vi "Bumper Start BAP7.vi"(11 "Port (Port 1)":T2=1 items=["Port 1", "Port 2", "Port 3", "Port 4"]) -> (3 "BrickReference out":T1)   [LabVIEW 2014]
doc: "Bumper Start BAP7\n\nPlays a note when front sensor is pressed. (Idle State)\n\nBeverly Abadines\nPHY 350\nBAP7"
uses:
  <vilib>/NXT/Block Support/NXT_InputPort.ctl
  <vilib>/NXT/Subs/LVHSConnector.ctl
  <vilib>/NXT/LegoClasses/BrickReference/BrickReference.lvclass
  <vilib>/NXT/Dual Mode Library/Sound/PlayC.vi
panel:
  # "Bumper Start"
  # "Beverly Abadines\nPhys 350\nP7"
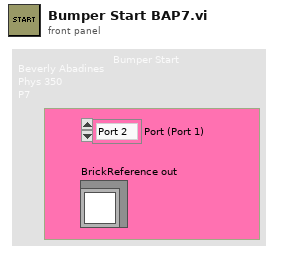
[diagram p1: front panel]
types:
  T1 = typedef "LVHSConnector.ctl" = refnum<class "BrickReference.lvclass">
  T2 = typedef "NXT_InputPort.ctl" = u32
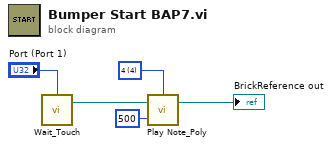
[diagram p0: block diagram]
diagram:
  w1 = u16 4 items=["3"=3, "4"=4, "5"=5, "6"=6, "7"=7] ("Octave")
  n1 = call <vilib>:"Wait_Touch.vi"("Port (Port 1)"="Port (Port 1)") -> ("NXT/EV3"=w3:T1)  [unwired: 3 in]
  n2 = call-poly <vilib>:"Play Note_Poly.vi"("Duration (500 ms)"=u16 500, "NXT/EV3"=w3, "Octave"=w1) -> ("NXT/EV3"=→"BrickReference out":T1)  [unwired: 1 in]
